vi "List All Topics.vi"(11 "TopicLookupTable":refnum<data-value>) -> (2 "Topic List":string[][](array[string]))   [LabVIEW 2015, in "Mediator.lvlib" / "TopicLookupTable.lvclass"]
doc: "<License>\nCopyright © 2017 Composed Systems, LLC | All rights reserved\nwww.composed.io\n\nAuthor: Ethan Stern <ethan.stern@composed.io>\n\nThis software is provided \"AS IS\" WITHOUT WARRANTIES, either express or implied, AND IS FOR EDUCATIONAL PURPOSES ONLY.\n</License>"
uses:
  TopicLookupTable.lvclass
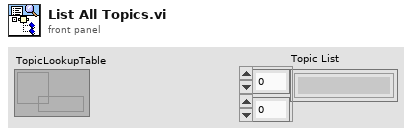
[diagram p1: front panel]
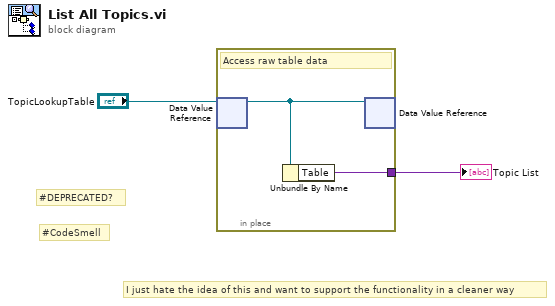
[diagram p0: block diagram]
diagram:
  # "#CodeSmell"
  # "I just hate the idea of this and want to support the functionality in a cleaner way"
  # "#DEPRECATED?"
  n1 = in-place {
    in-place-border: [w4] -> w1
    # "Access raw table data"
    n2 = in-place-dvr #1("TopicLookupTable") -> (w3:refnum<class "TopicLookupTable.lvclass">)  [unwired: 1 out]
    n3 = Unbundle By Name(w3) -> ("Table"=w4:variant)
    n4 = in-place-dvr #1(w3) -> ()  [unwired: 2 out]
  }
  "Topic List" <- w1
